vi "Latch(1).vi"() -> ()   [LabVIEW 2011]
panel:
  out "Input":bool
  out "Output":bool
  in  "OK Button":bool
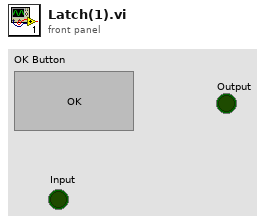
[diagram p1: front panel]
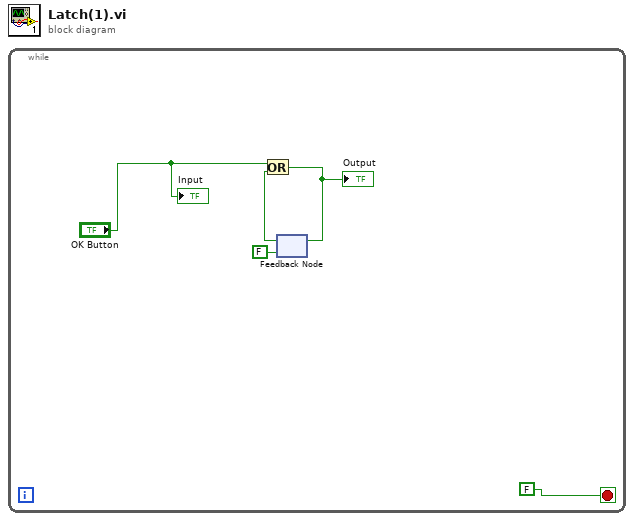
[diagram p0: block diagram]
diagram:
  n1 = while {
    stop <- FALSE stop-if-true
    n2 = feedback #1(FALSE) -> (w4:bool)
    n3 = Or(x="OK Button", y=w4) -> (x .or. y?=w5:bool)
    "Output" <- w5
    n4 = feedback-in #1(w5) -> ()
    "Input" <- "OK Button"
  }
